vi "test - Fit VI to Window.vi"   [LabVIEW 2017]
uses:
  user.lib/NEVSTOP-Programming-Palette/Dialog & Interface/Fit VI window to Visible Content.vi
  user.lib/NEVSTOP-Programming-Palette/Dialog & Interface/Fit VI window to Content.vi
  user.lib/NEVSTOP-Programming-Palette/Dialog & Interface/Fit VI window to Largest Dec.vi
  user.lib/NEVSTOP-Programming-Palette/Dialog & Interface/Fit VI window to Caller Center.vi
  user.lib/NEVSTOP-Programming-Palette/Dialog & Interface/Fit VI window to Pane Center.vi
  user.lib/NEVSTOP-Programming-Palette/Dialog & Interface/Fit VI window to Panel Center.vi
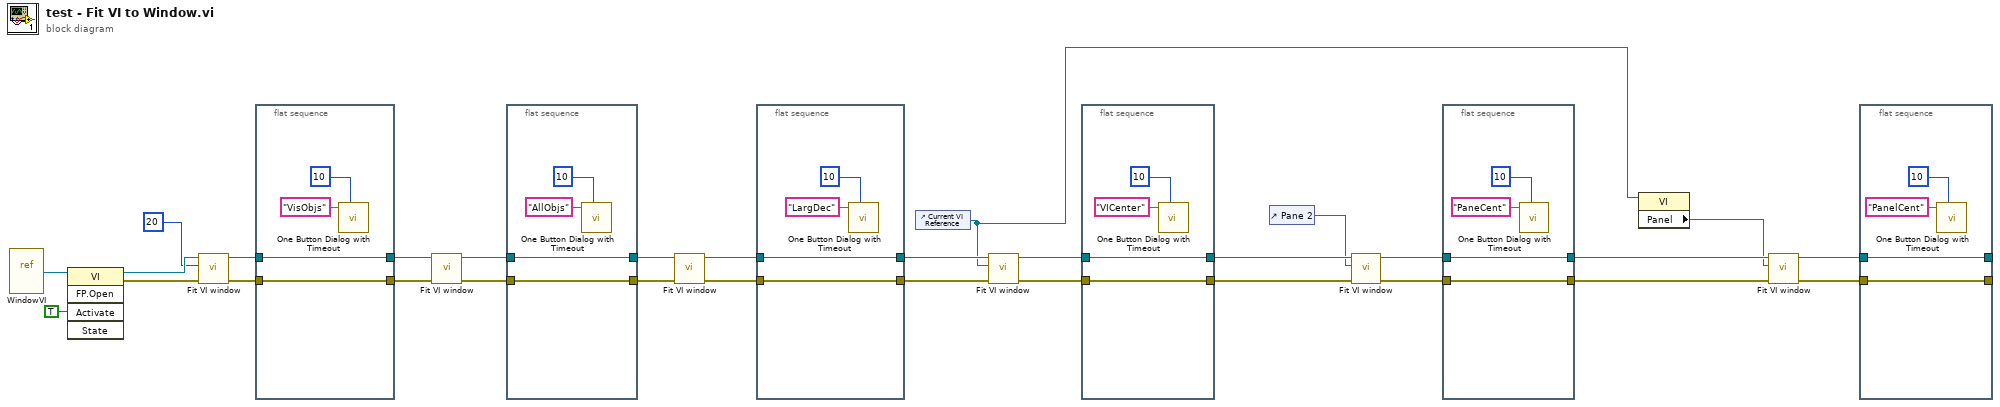
[diagram p0: block diagram]
diagram:
  n1 = vi-ref "WindowVI.vi"() -> (w30:refnum<vi>)
  n2 = invoke class="VI" method="FP.Open"(reference=w30, "Activate"=TRUE ("Activate?")) -> (reference out=w27:refnum<vi>, error out=w28:errorcluster)  [unwired: 3 in, 3 out]
  n3 = call-poly "Fit VI window.vi"("error in (no error)"=w28, "border spacing (2 px)"=20, "VI Ref (calling VI)"=w27) -> ("error out"=w24:errorcluster, "dup VI Ref"=w23:refnum<vi>)  [unwired: 3 in]
  n4 = flat-sequence {
    tunnel: [w32] -> w25
    tunnel: w24 -> [w32]
    tunnel: w23 -> [w31]
    tunnel: [w31] -> w22
    frame #0 {
      n5 = call "One Button Dialog with Timeout.vi"("message"="VisObjs", "Btn Timeout(-1 s)"=10) -> ()  [unwired: 7 in, 1 out]
    }
  }
  n6 = call-poly "Fit VI window.vi"("error in (no error)"=w25, "VI Ref (calling VI)"=w22) -> ("error out"=w19:errorcluster, "dup VI Ref"=w18:refnum<vi>)  [unwired: 4 in]
  n7 = flat-sequence {
    tunnel: [w36] -> w20
    tunnel: w19 -> [w36]
    tunnel: w18 -> [w35]
    tunnel: [w35] -> w21
    frame #0 {
      n8 = call "One Button Dialog with Timeout.vi"("message"="AllObjs", "Btn Timeout(-1 s)"=10) -> ()  [unwired: 7 in, 1 out]
    }
  }
  n9 = call-poly "Fit VI window.vi"("error in (no error)"=w20, "VI Ref (calling VI)"=w21) -> ("error out"=w15:errorcluster, "dup VI Ref"=w14:refnum<vi>)  [unwired: 4 in]
  n10 = flat-sequence {
    tunnel: [w40] -> w17
    tunnel: w15 -> [w40]
    tunnel: w14 -> [w39]
    tunnel: [w39] -> w16
    frame #0 {
      n11 = call "One Button Dialog with Timeout.vi"("message"="LargDec", "Btn Timeout(-1 s)"=10) -> ()  [unwired: 7 in, 1 out]
    }
  }
  n12 = control-ref of="Current VI Reference"() -> (w2:refnum<vi>)
  n13 = call-poly "Fit VI window.vi"("Error In"=w17, "Background VI Ref (Callee's Caller)"=w2, "VI Ref (calling VI)"=w16) -> ("Error Out"=w11:errorcluster, "dup VI Ref"=w10:refnum<vi>)  [unwired: 3 in]
  n14 = flat-sequence {
    tunnel: [w44] -> w12
    tunnel: w11 -> [w44]
    tunnel: w10 -> [w43]
    tunnel: [w43] -> w13
    frame #0 {
      n15 = call "One Button Dialog with Timeout.vi"("message"="VICenter", "Btn Timeout(-1 s)"=10) -> ()  [unwired: 7 in, 1 out]
    }
  }
  n16 = control-ref of="Pane 2"() -> (w9:refnum<vi>)
  n17 = call-poly "Fit VI window.vi"("Error In"=w12, "Pane Ref"=w9, "VI Ref (calling VI)"=w13) -> ("Error Out"=w8:errorcluster, "dup VI Ref"=w7:refnum<vi>)  [unwired: 3 in]
  n18 = flat-sequence {
    tunnel: [w48] -> w4
    tunnel: w8 -> [w48]
    tunnel: w7 -> [w47]
    tunnel: [w47] -> w3
    frame #0 {
      n19 = call "One Button Dialog with Timeout.vi"("message"="PaneCent", "Btn Timeout(-1 s)"=10) -> ()  [unwired: 7 in, 1 out]
    }
  }
  n20 = property class="VI"(reference=w2) -> ("Panel"=w1:refnum<vi>)  [unwired: 1 in, 2 out]
  n21 = call-poly "Fit VI window.vi"("Error In"=w4, "Panel Ref"=w1, "VI Ref (calling VI)"=w3) -> ("Error Out"=w5:errorcluster, "dup VI Ref"=w6:refnum<vi>)  [unwired: 3 in]
  n22 = flat-sequence {
    tunnel: [w52] -> _
    tunnel: w5 -> [w52]
    tunnel: w6 -> [w51]
    tunnel: [w51] -> _
    frame #0 {
      n23 = call "One Button Dialog with Timeout.vi"("message"="PanelCent", "Btn Timeout(-1 s)"=10) -> ()  [unwired: 7 in, 1 out]
    }
  }
